vi "Get_Maximal_Length_of_Subtracks(101-11)-1.vi"(1 "[IN] Subtracks":T1(array[cluster]), 2 "[IN] Number of costs":i32) -> (0 "[OUT] Maximal Length":i32)   [LabVIEW 2013]
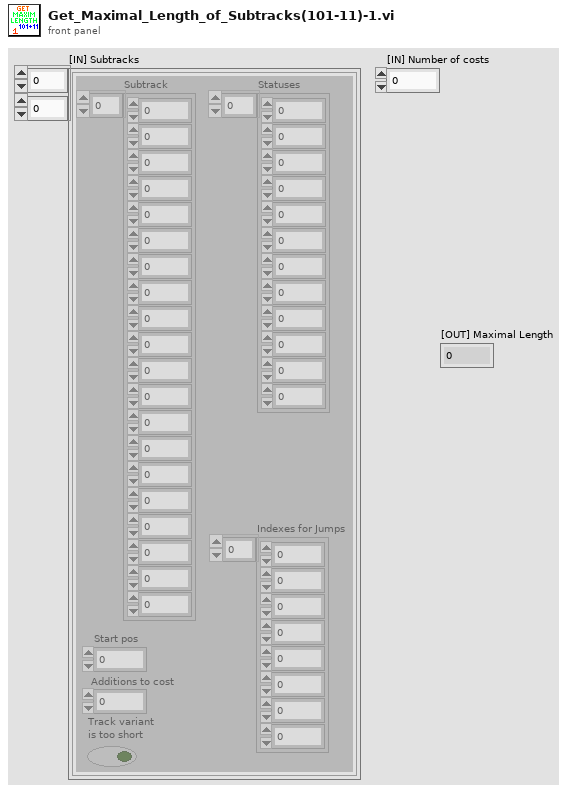
[diagram p1: front panel]
types:
  T1 = cluster{"Subtrack":dbl[], "Statuses":i16[], "Start pos":i32, "Additions to cost":i32, "Track variant \nis too short":bool, "Indexes for Jumps":i32[]}[][]
  T2 = cluster{"Subtrack":dbl[], "Statuses":i16[], "Start pos":i32, "Additions to cost":i32, "Track variant \nis too short":bool, "Indexes for Jumps":i32[]}[]
  T3 = cluster{"Subtrack":dbl[], "Statuses":i16[], "Start pos":i32, "Additions to cost":i32, "Track variant \nis too short":bool, "Indexes for Jumps":i32[]}
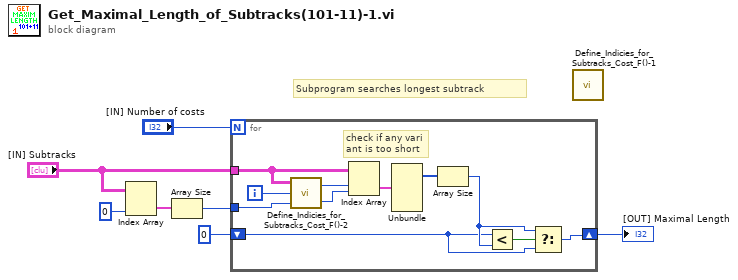
[diagram p0: block diagram]
diagram:
  # "Subprogram searches longest subtrack"
  n1 = Index Array(array="[IN] Subtracks", index (col)=0 ("disabled index (col)")) -> (element=w4:T2)  [unwired: 1 in]
  n2 = Array Size(array=w4) -> (size(s)=w2:i32)
  n3 = for {
    N: "[IN] Number of costs" -> [_]
    tunnel: "[IN] Subtracks" -> [w12]
    shift-right: [w14] -> w6
    shift-left: 0 -> [w15]
    tunnel: w2 -> [w10]
    i -> [w11]
    # "check if any vari\nant is too short"
    n4 = call "Define_Indicies_for_Subtracks_Cost_F()-2.vi"("[IN] Number of Rows"=w10, "[IN] Current index"=w11, "[IN] Subtracks"=w12) -> ("[OUT] Column \n# for Subtrack"=w8:i32, "[OUT] Row # \nfor Subtrack"=w9:i32)
    n5 = Index Array(array=w12, index (row)=w9, index (col)=w8) -> (element=w18:T3)
    n6 = Unbundle(w18) -> ("Statuses"=w13:i16[])  [unwired: 5 out]
    n7 = Array Size(array=w13) -> (size(s)=w16:i32)
    n8 = Less?(x=w15, y=w16) -> (x < y?=w17:bool)
    n9 = Select(t=w16, s=w17, f=w15) -> (s? t:f=w14:i32)
  }
  "[OUT] Maximal Length" <- w6
  n10 = call "Define_Indicies_for_Subtracks_Cost_F()-1.vi"() -> ()  [unwired: 2 in, 2 out]
